vi "Write DenuderBypass.vi"(8 "error in (no error)":errorcluster, 10 "DenuderBypass":bool, 11 "xData in":refnum<class "xData.lvclass">) -> (0 "error out":errorcluster, 3 "xData out":refnum<class "xData.lvclass">)   [LabVIEW 2014, in "xData.lvclass"]
uses:
  xData.lvclass
  xData.lvclass/xData.ctl
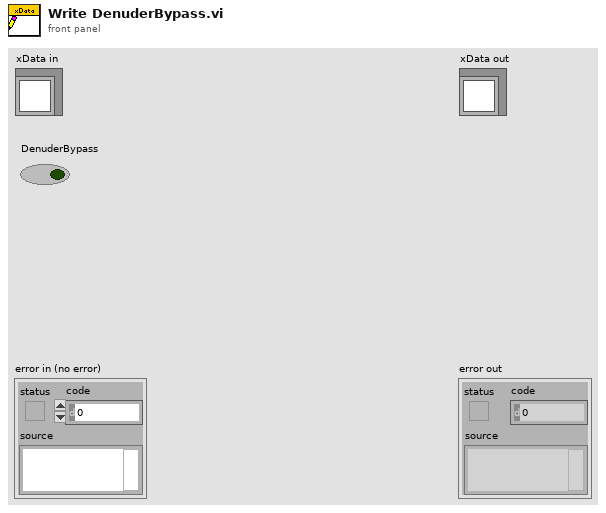
[diagram p1: front panel]
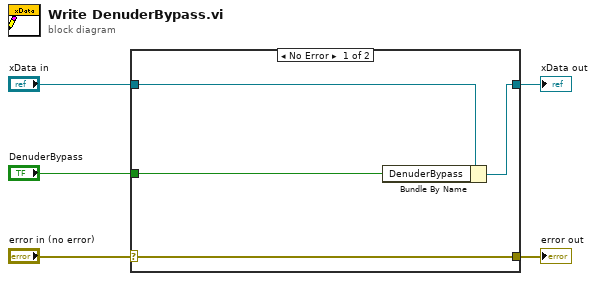
[diagram p0: block diagram]
diagram:
  n1 = case shown="No Error" "error in (no error)" {
    selector: "error in (no error)" -> [w9 w10]
    tunnel: [w9 w10] -> w4
    tunnel: [w7 w11] -> w2
    tunnel: "xData in" -> [w8 w11]
    tunnel: "DenuderBypass" -> [w6 _]
    frame No Error {
      n2 = Bundle By Name(cluster=w8, "DenuderBypass"=w6) -> (w7:refnum<class "xData.lvclass">)
    }
    frame Error {
    }
  }
  "error out" <- w4
  "xData out" <- w2
